vi "Test_Single folder menu refresh.vi"() -> ()   [LabVIEW 2019]
uses:
  Build/Menu.AutoMenuCreator.lvlibp
panel:
  out "error out":errorcluster
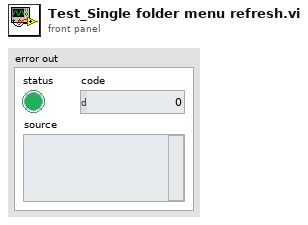
[diagram p1: front panel]
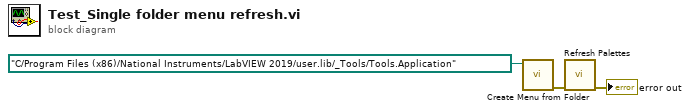
[diagram p0: block diagram]
diagram:
  n1 = call "Create Menu from Folder.vi"("Target Folder"=path "C:/Program Files (x86)/National Instruments/LabVIEW 2019/user.lib/_Tools/Tools.Application") -> ("error out"=w3:errorcluster)  [unwired: 10 in]
  n2 = call "Refresh Palettes.vi"("error in (no error)"=w3) -> ("error out"=→"error out":errorcluster)  [unwired: 10 in]
